vi "Determine Warnings - Reusable subVIs.vi"(6 "High":dbl, 7 "wind":dbl, 8 "error in (no error)":errorcluster, 9 "Low":dbl, 10 "Hi":dbl, 11 "Temp":dbl) -> (0 "error out":errorcluster, 1 "Stop":bool, 2 "text":string)   [LabVIEW 2010]
doc: "This is an exercise VI used in LabVIEW Core II. It is an example of inherited code that needs to be improved. Improve the VI for readability and maintainability, without changing the functionality."
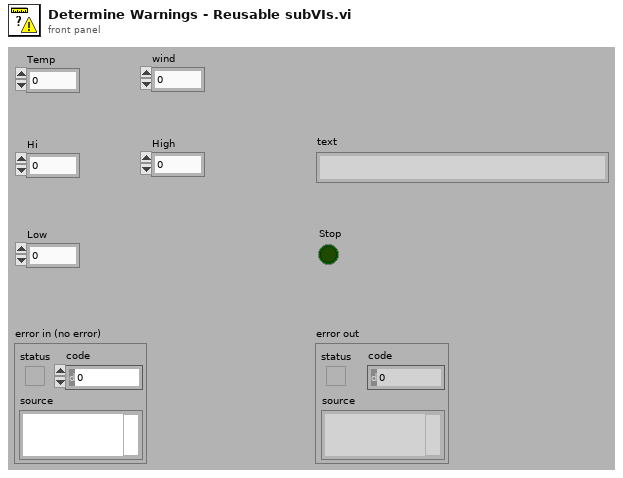
[diagram p1: front panel]
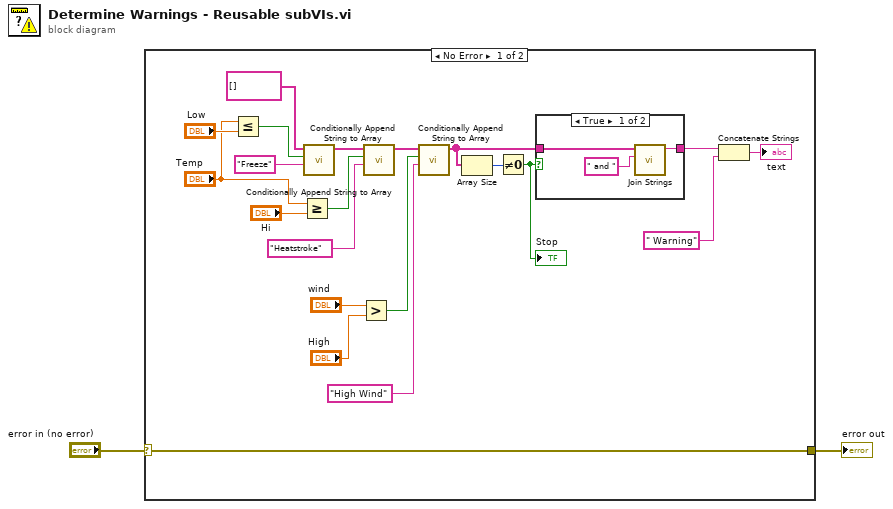
[diagram p0: block diagram]
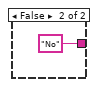
[diagram p2: hidden frame]
diagram:
  n1 = case shown="No Error" "error in (no error)" {
    selector: "error in (no error)" -> [w3 w28]
    tunnel: [w3 w28] -> w1
    frame No Error {
      n2 = Less Or Equal?(x="Temp", y="Low") -> (x <= y?=w18:bool)
      n3 = Greater Or Equal?(x="Temp", y="Hi") -> (x >= y?=w13:bool)
      n4 = call "Conditionally Append String to Array.vi"("Text to add to array"="Freeze", "Append?"=w18, "String array in"=string[] []) -> ("String array out"=w15:string[])  [unwired: 8 out]
      n5 = Greater?(x="wind", y="High") -> (0:w11:bool)
      n6 = call "Conditionally Append String to Array.vi"("Text to add to array"="Heatstroke", "Append?"=w13, "String array in"=w15) -> ("String array out"=w14:string[])  [unwired: 8 out]
      n7 = call "Conditionally Append String to Array.vi"("Text to add to array"="High Wind", "Append?"=w11, "String array in"=w14) -> ("String array out"=w9:string[])  [unwired: 8 out]
      n8 = Array Size(array=w9) -> (size(s)=w8:i32)
      n9 = Not Equal To 0?(x=w8) -> (x != 0?=w7:bool)
      "Stop" <- w7
      n10 = case shown="True" w7 {
        tunnel: [w25 "No" ("f")] -> w5
        tunnel: w9 -> [w26 _]
        frame True {
          n11 = call "Join Strings.vi"("Delimeter (\", \")"=" and " ("delimiter (Tab)"), "Strings"=w26) -> ("Joined string"=w25:string)  [unwired: 9 out]
        }
        frame False {
        }
      }
      n12 = Concatenate Strings(w5, " Warning" ("string")) -> (→"text":string)
    }
    frame Error {
    }
  }
  "error out" <- w1
